vi "zlgcan_demo_DTU.vi"() -> ()   [LabVIEW 2018]
uses:
  data_type/ZCAN_InitCAN_setting_DTU.ctl
panel:
  in  "是否使用电阻":u8(ring)=1 items=["不使用终端电阻", "使用终端电阻"]
  in  "工作模式":u8(ring)=1 items=["正常"=1, "只听"=0]
  in  "自定义波特率字符输入":string
  in  "使用自定义波特率？":bool
  in  "波特率":u32(ring)=500000 items=["1Mbps"=1000000, "800kbps"=800000, "500kbps"=500000, "250kbps"=250000, "125kbps"=125000, "100kbps"=100000, "50kbps"=50000]
  in  "通道索引":u32(ring) items=["0", "1", "2", "3"]
  in  "设备索引":u32(ring) items=["0", "1", "2", "3"]
  in  "设备类型":u32(ring)=32 items=["PCI-9810"=2, "USBCAN-II"=4, "USBCAN-E-U"=20, "CANDTU-200 XX"=32, "CANDTU_100UR"=37, "USBCANFD-100U"=42, "USBCANFD-200U"=41, "PCIE-CANFD-100U"=38, "PCIE-CANFD-200U"=39, "PCIE-CANFD-400U"=40, "云设备"=46]
  in  "开启CAN":bool
  in  "stop":bool
  in  "ID":u32 format="0x%08x"
  in  "数据长度(最大8字节)":u8=8 max=8
  in  "Data Byte 8":u8 caption="data88" format="%.0x"
  in  "Data Byte 7":u8 caption="data7" format="%.0x"
  in  "Data Byte 6":u8 caption="data6" format="%.0x"
  in  "Data Byte 5":u8 caption="data5" format="%.0x"
  in  "Data Byte 4":u8 caption="data4" format="%.0x"
  in  "Data Byte 3":u8 caption="data3" format="%.0x"
  in  "Data Byte 2":u8 caption="data2" format="%.0x"
  in  "Data Byte 1":u8 caption="data1" format="%.0x"
  in  "帧格式":u32(ring) items=["数据帧", "远程帧"]
  in  "发送方式":u32(ring) items=["正常发送", "单次发送", "自发自收", "单次自发自收"]
  in  "帧类型":u32(ring) items=["标准帧", "扩展帧"]
  in  "每次发送帧数":u32=1
  in  "发送":bool
  out "error out":errorcluster caption="错误输出"
  in  "DTU系列初始化参数":T1
  out "can_index_handle(out)":u32
  out "Device_handle(out)":u32
  out "已接收帧数":u32
  out "接收字符串显示":string caption="String"
  # "停止程序前，需要先关闭CAN卡"
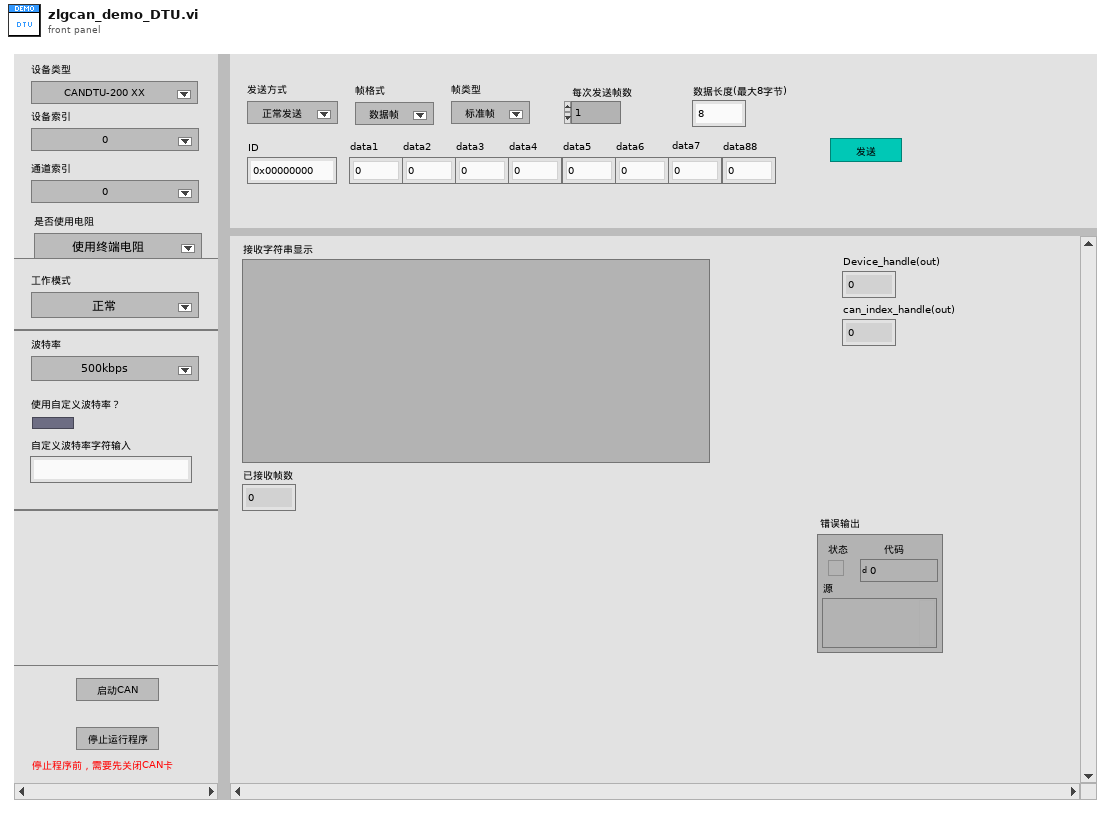
[diagram p1: front panel]
types:
  T1 = typedef "ZCAN_InitCAN_setting_DTU.ctl" = cluster{"baudrate":u32, "baud_rate_custom？":bool, "RateCustom":string, "work_mode":u32}
  T2 = cluster{"[0]":u8, "[1]":u8, "[2]":u8, "[3]":u8, "[4]":u8, "[5]":u8, "[6]":u8, "[7]":u8}
  T3 = cluster{u32, u8, u8, u8, u8, cluster{"[0]":u8, "[1]":u8, "[2]":u8, "[3]":u8, "[4]":u8, "[5]":u8, "[6]":u8, "[7]":u8}, u64}[]
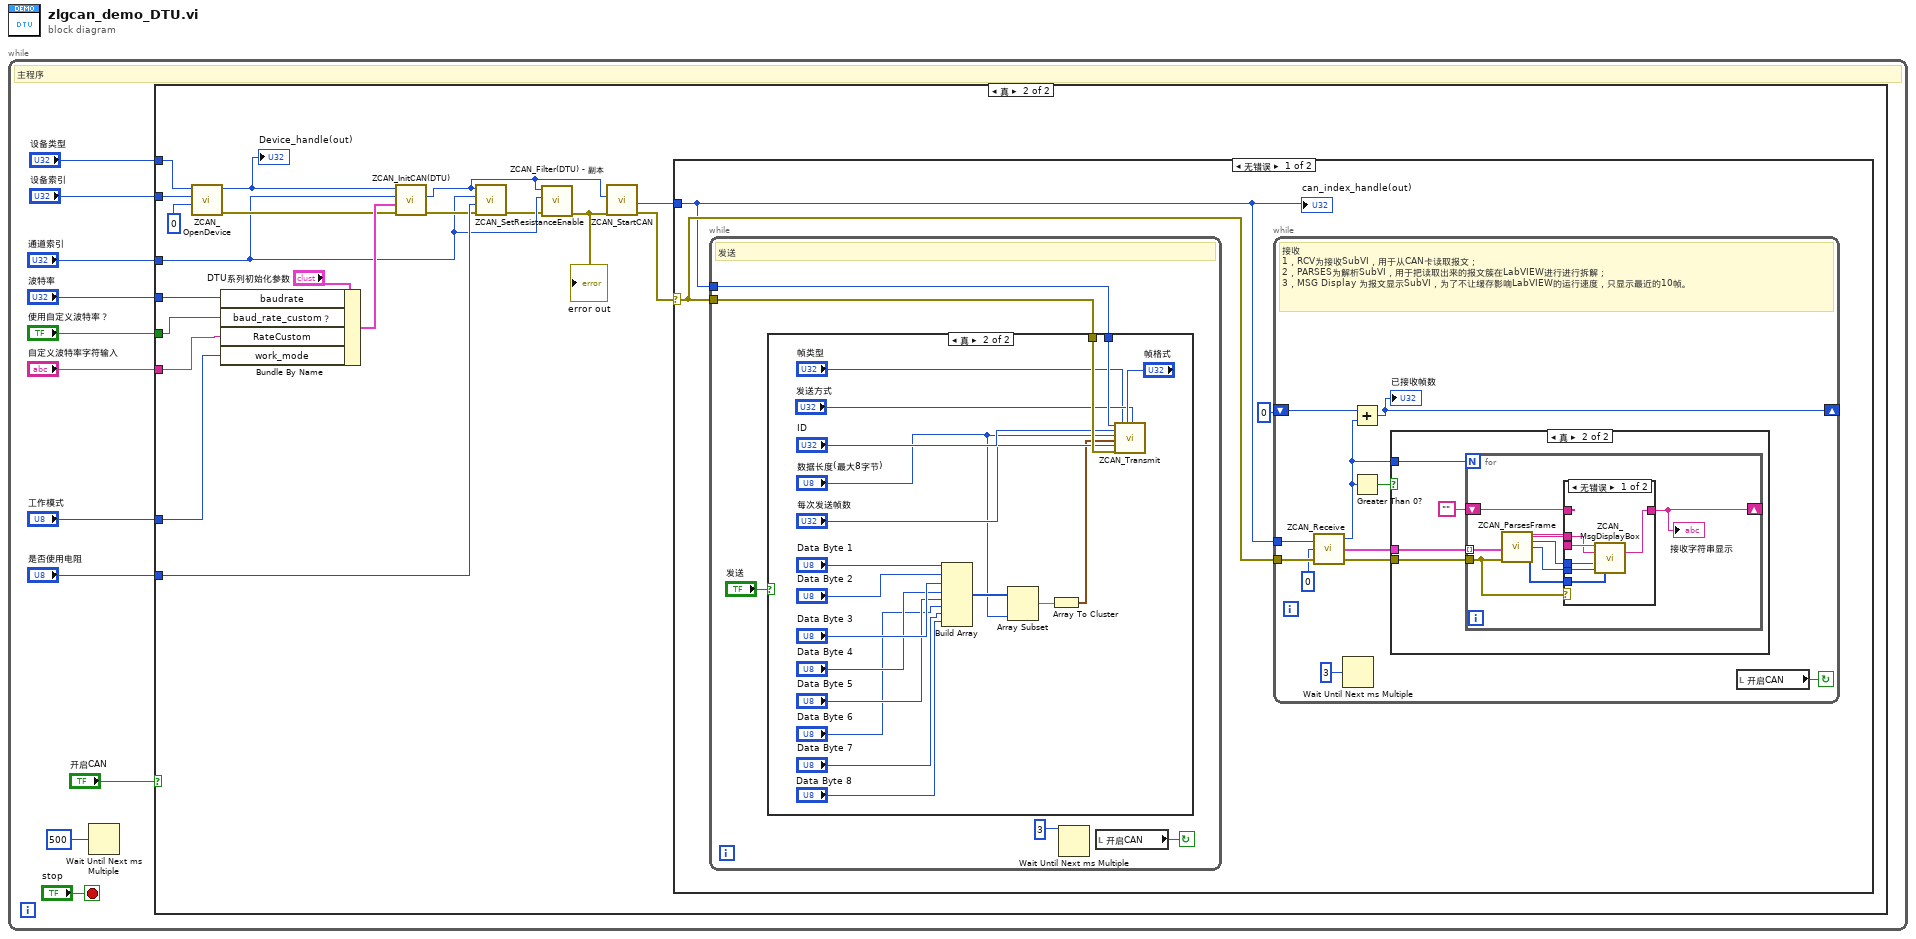
[diagram p0: block diagram]
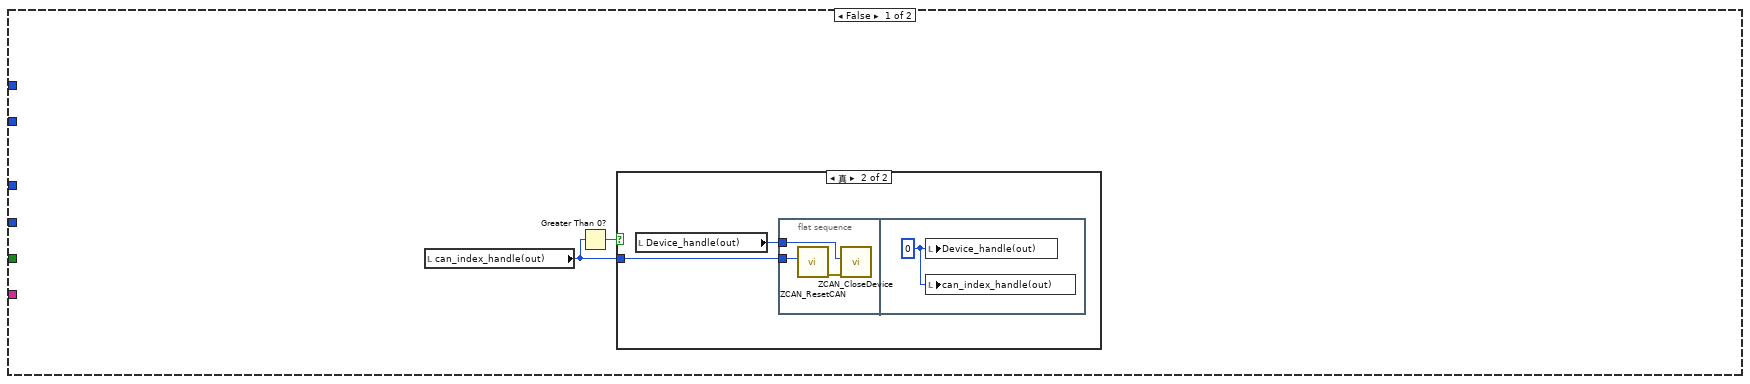
[diagram p2: hidden frame]
diagram:
  n1 = while {
    stop <- "stop" stop-if-true
    # "主程序"
    n2 = Wait Until Next ms Multiple(millisecond multiple=u32 500) -> ()  [unwired: 1 out]
    n3 = case shown="真" "开启CAN" {
      tunnel: "通道索引" -> [_ w24]
      tunnel: "波特率" -> [_ w31]
      tunnel: "使用自定义波特率？" -> [_ w30]
      tunnel: "自定义波特率字符输入" -> [_ w29]
      tunnel: "工作模式" -> [_ w28]
      tunnel: "设备类型" -> [_ w36]
      tunnel: "设备索引" -> [_ w37]
      tunnel: "是否使用电阻" -> [_ w33]
      frame False {
        # "关闭CAN卡"
        n4 = local read "can_index_handle(out)"() -> (w12:u32)
        n5 = Greater Than 0?(x=w12) -> (x > 0?=w13:bool)
        n6 = case shown="真" w13 {
          tunnel: w12 -> [_ w15]
          frame False {
          }
          frame True {
            n7 = local read "Device_handle(out)"() -> (w14:u32)
            n8 = flat-sequence {
              tunnel: w15 -> [w17]
              tunnel: w14 -> [w16]
              frame #0 {
                n9 = call "ZCAN_ResetCAN.vi"("can_handle"=w17) -> ("error out"=w18:errorcluster)  [unwired: 9 in, 1 out]
                n10 = call "ZCAN_CloseDevice.vi"("error in (no error)"=w18, "device_handle"=w16) -> ()  [unwired: 8 in, 2 out]
              }
              frame #1 {
                w19 = u32 0 ("can_index_handle(out)")
                n11 = local write "Device_handle(out)"(w19) -> ()
                n12 = local write "can_index_handle(out)"(w19) -> ()
              }
            }
          }
        }
      }
      frame True {
        n13 = call "ZCAN_OpenDevice.vi"("reserved"=0, "device_index"=w37, "device_type"=w36) -> ("error out"=w26:errorcluster, "DEVICE_HANDLE"=w21:u32)  [unwired: 7 in]
        "Device_handle(out)" <- w21
        n14 = Bundle By Name(cluster="DTU系列初始化参数", "baudrate"=w31, "baud_rate_custom？"=w30, "RateCustom"=w29, "work_mode"=w28) -> (w27:T1)
        n15 = call "ZCAN_InitCAN(DTU).vi"("error in (no error)"=w26, "DTU系列初始化参数"=w27, "can_index"=w24, "device_hande"=w21) -> ("error out"=w25:errorcluster, "can_index_handle"=w20:u32)  [unwired: 2 in]
        n16 = call "ZCAN_SetResistanceEnable.vi"("error in (no error)"=w25, "enable"=w33, "can_index"=w24, "can_index_handle"=w20) -> ("error out"=w23:errorcluster)  [unwired: 7 in]
        n17 = call "ZCAN_Filter(DTU) - 副本.vi"("error in (no error)"=w23, "can_index"=w24, "device_handle"=w20) -> ("error out"=w22:errorcluster)  [unwired: 7 in]
        "error out" <- w22
        n18 = call "ZCAN_StartCAN.vi"("error in (no error)"=w22, "can_index_handle"=w20) -> ("error out"=w34:errorcluster, "can_index_handle(out)"=w35:u32)  [unwired: 7 in, 1 out]
        n19 = case shown="无错误" w34 {
          selector: w34 -> [w40 _]
          tunnel: w35 -> [w39 _]
          frame No Error {
            n20 = while {
              tunnel: w39 -> [w75]
              tunnel: w40 -> [w73]
              stop <- w74 continue-if-true
              # "发送"
              n21 = case shown="真" "发送" {
                tunnel: w75 -> [_ w96]
                tunnel: w73 -> [_ w95]
                frame False {
                }
                frame True {
                  n22 = Build Array("Data Byte 1", "Data Byte 2", "Data Byte 3", "Data Byte 4", "Data Byte 5", "Data Byte 6", "Data Byte 7", "Data Byte 8") -> (w82:u8[])
                  n23 = Array Subset(array=w82, length="数据长度(最大8字节)") -> (w80:u8[])  [unwired: 1 in]
                  n24 = Array To Cluster(array=w80) -> (cluster=w79:T2)
                  n25 = call "ZCAN_Transmit.vi"("can_index_handle"=w96, "ID"="ID", "数据长度"="数据长度(最大8字节)", "DATA"=w79, "每次发送帧数"="每次发送帧数", "error in (no error)"=w95, "帧类型"="帧类型", "帧格式"="帧格式", "发送方式"="发送方式") -> ()  [unwired: 10 in, 1 out]
                }
              }
              n26 = Wait Until Next ms Multiple(millisecond multiple=u32 3) -> ()  [unwired: 1 out]
              n27 = local read "开启CAN"() -> (w74:bool)
            }
            n28 = while {
              tunnel: w40 -> [w49]
              tunnel: w39 -> [w47]
              shift-right: [w50] -> _
              shift-left: 0 -> [w51]
              stop <- w42 continue-if-true
              # "接收\n1，RCV为接收SubVI，用于从CAN卡读取报文；\n2，PARSES为解析SubVI，用于把读取出来的报文簇在LabVIEW进行进行拆解；\n3，MSG Display 为报文显示SubVI，为了不让缓存影响LabVIEW的运行速度，只显示最近的10帧。"
              n29 = call "ZCAN_Receive.vi"("error in (no error)"=w49, "type"=u8 0, "can_handle"=w47) -> ("error out"=w45:errorcluster, "Receive"=w46:T3, "Receive_Num"=w44:u32)
              n30 = Wait Until Next ms Multiple(millisecond multiple=u32 3) -> ()  [unwired: 1 out]
              n31 = Add(x=w51, y=w44) -> (x+y=w50:u32)
              "已接收帧数" <- w50
              n32 = Greater Than 0?(x=w44) -> (x > 0?=w43:bool)
              n33 = case shown="真" w43 {
                tunnel: w44 -> [_ w56]
                tunnel: w46 -> [_ w55]
                tunnel: w45 -> [_ w54]
                frame False {
                }
                frame True {
                  n34 = for {
                    N: w56 -> [_]
                    tunnel: w55 -> [w63] mode=indexing
                    tunnel: w54 -> [w62]
                    shift-right: [w65] -> _
                    shift-left: "" -> [w64]
                    n35 = call "ZCAN_ParsesFrame.vi"("ZCAN_Receive_Data"=w63, "error in (no error)"=w62) -> ("帧格式"=w57:string, "帧类型"=w58:string, "ID"=w59:u32, "data_len"=w61:u8, "data"=w60:u8[])  [unwired: 8 in, 1 out]
                    n36 = case shown="无错误" w62 {
                      tunnel: [w71 w72] -> w65
                      tunnel: w64 -> [_ w72]
                      tunnel: w61 -> [w70 _]
                      tunnel: w60 -> [w69 _]
                      tunnel: w59 -> [w68 _]
                      tunnel: w58 -> [w67 _]
                      tunnel: w57 -> [w66 _]
                      frame No Error {
                        n37 = call "ZCAN_MsgDisplayBox.vi"("帧类型"=w67, "ID"=w68, "帧格式"=w66, "Message Data"=w69, "data_len"=w70) -> ("Output String"=w71:string)  [unwired: 10 in]
                      }
                      frame Error {
                      }
                    }
                    "接收字符串显示" <- w65
                  }
                }
              }
              n38 = local read "开启CAN"() -> (w42:bool)
            }
            "can_index_handle(out)" <- w39
          }
          frame Error {
          }
        }
      }
    }
  }
